vi "DAQmxStrain.vi"() -> ()   [LabVIEW 2010]
uses:
  <vilib>/DAQmx/read.llb/DAQmx Read.vi
  <vilib>/DAQmx/read.llb/DAQmx Read (Analog 1D Wfm NChan NSamp).vi
  <vilib>/Waveform/WDTOps.llb/WDT Get XY Value DBL.vi
  <vilib>/daqmx/miscellaneous.llb/DAQmx Fill In Error Info.vi
panel:
  out "应变值":dbl format="%0.2f"
  out "应变数据":waveform(dbl)[](graph)
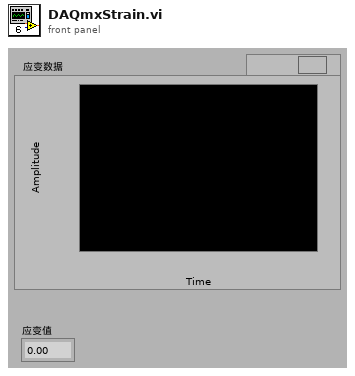
[diagram p1: front panel]
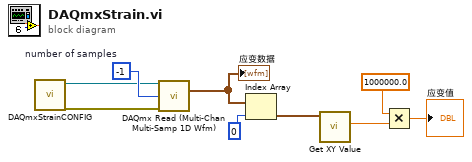
[diagram p0: block diagram]
diagram:
  w9 = -1  # number of samples
  n1 = call "DAQmxStrainCONFIG.vi"() -> ("error out"=w7:errorcluster, "task out"=w8:refnum<k21>)  [unwired: 10 in]
  n2 = call-poly "DAQmx Read (Multi-Chan Multi-Samp 1D Wfm).vi"("task/channels in"=w8, "number of samples per channel"=w9, "error in"=w7) -> ("data"=w6:waveform(dbl)[])  [unwired: 10 in, 2 out]
  "应变数据" <- w6
  n3 = Index Array(array=w6, index=0) -> (element=w4:waveform(dbl))
  n4 = call-poly <vilib>:"Get XY Value.vi"("waveform in"=w4) -> ("Y value"=w3:dbl)  [unwired: 6 in, 4 out]
  n5 = Multiply(x=1000000.0, y=w3) -> (x*y=→"应变值":dbl)
